vi "GenerateFileHeader.vi"() -> (3 "Position File Header":string[](array[string]))   [LabVIEW 2012]
doc: "SciScan 1.2 160622"
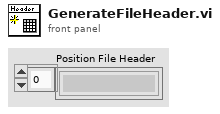
[diagram p1: front panel]
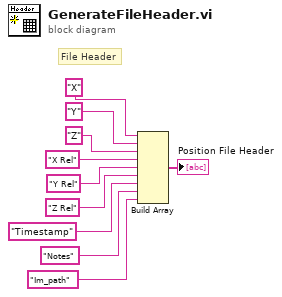
[diagram p0: block diagram]
diagram:
  # "File Header"
  n1 = Build Array("X", "Y", "Z", "X Rel", "Y Rel", "Z Rel", "Timestamp", "Notes", "Im_path") -> (→"Position File Header":string[])
